vi "03 - 2D Picture.vi"() -> ()   [LabVIEW 2019]
uses:
  Shared/Direction--enum.ctl
  Shared/Selection--picture ring.ctl
  Shared/Pen Operation--enum.ctl
  <vilib>/Utility/cursorutil.llb/Set Cursor (Icon Pict).vi
  Grassfire 2D/Grassfire 2D.lvclass
  Grassfire/Grassfire.lvclass
  Shared/Shared.lvlib
panel:
  in  "Zoom":sgl(slide) scale=1.0..5.0
  in  "Tab Control":enum32{"Edit", "Solution"}(tab)
  in  "Tool":enum32{"Erase", "Pen", "Start", "End"}(radio)
  out "Maze":picture
  in  "Load File":bool
  in  "Save File":bool
  in  "Preset 1":bool
  in  "Pen Color":u32(colorbox)=15671808
  in  "Select Pen Attributes":T1={"Width"=6, "Style"=enum."Solid"} {"Width" scale=1.0..5.0}
  in  "Clear":bool
  in  "Selection":T2
  in  "Pen":T3
  in  "Calculate":bool
  in  "Heading":T4=enum."Down"
  out "Maze Solution":picture
  out "ms":u32
  out "Directions":T4[](array[typedef])
  out "Valid":bool
  in  "Calculate using Class in Maps":bool
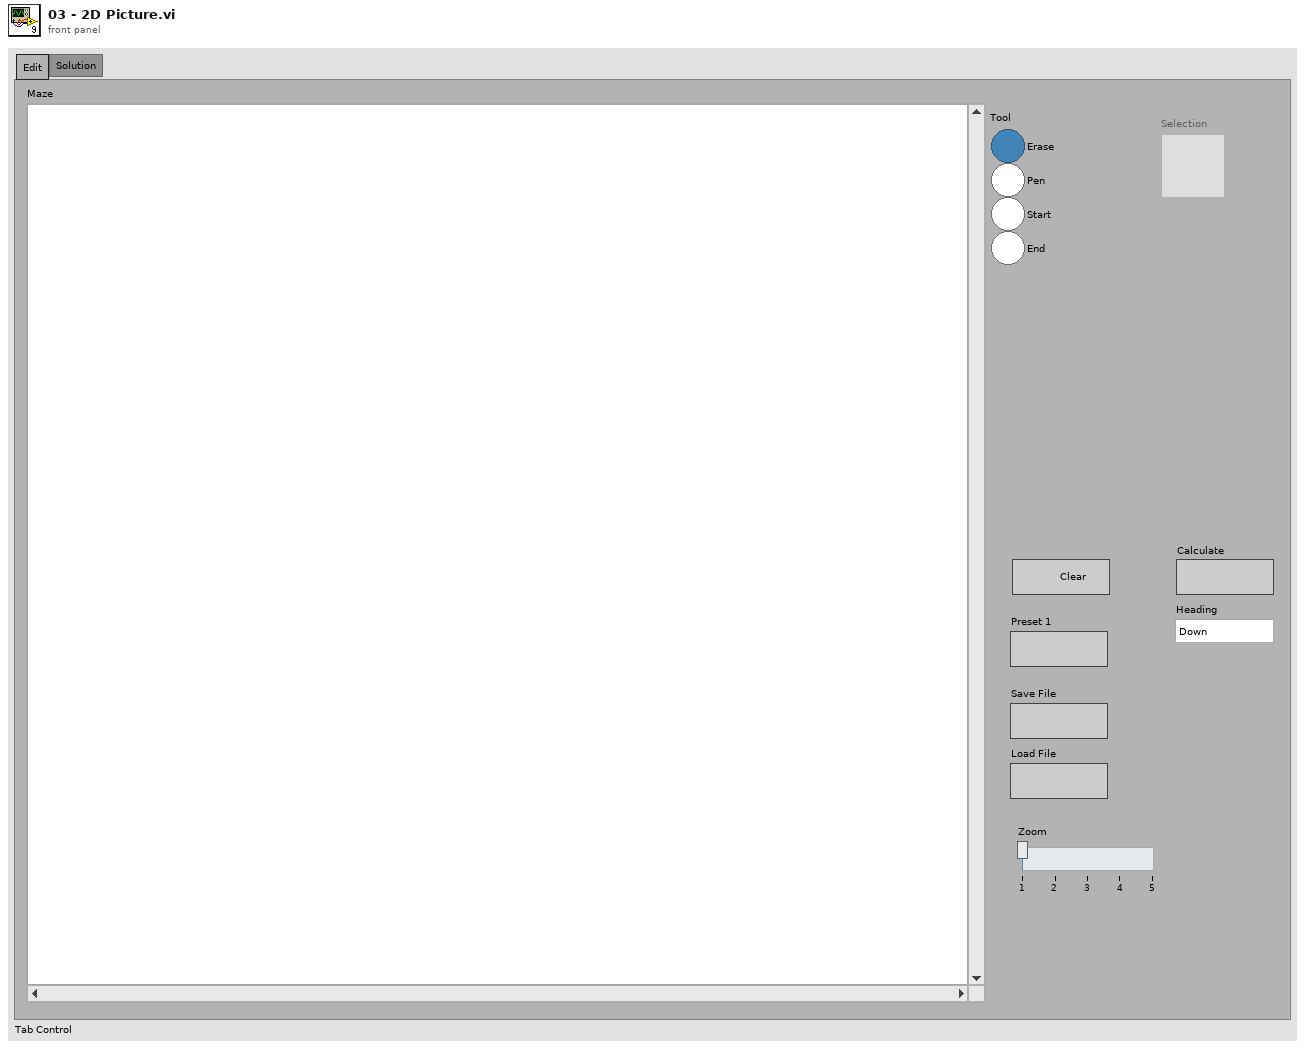
[diagram p1: front panel]
types:
  T1 = cluster{"Width":u16, "Style":enum32{"Solid", "Dash", "Dot", "DashDot", "DashDotDot"}}
  T2 = typedef "Shared.lvlib/Selection--picture ring.ctl" = i64
  T3 = typedef "Shared.lvlib/Pen Operation--enum.ctl" = enum32{"Point", "Free", "Straight Line", "Rectangle"}
  T4 = typedef "Shared.lvlib/Direction--enum.ctl" = enum16{"<Unknown>", "Right", "Down", "Left", "Up"}
  T5 = enum32{"Solid", "Dash", "Dot", "DashDot", "DashDotDot"}
  T6 = typedef "LVMouseTypeDef.ctl" = cluster{"Mouse Position":cluster{"X":i32, "Y":i32}, "Mouse Modifiers":cluster{"Button Down":bool, "Shift Mod":bool, "Menu Mod":bool, "Option Mod":bool}}
  T7 = typedef "imagedata.ctl" = cluster{"image type":i32, "image depth":i32, "image":u8[], "mask":u8[], "colors":u32[], "Rectangle":cluster{"left":i16, "top":i16, "right":i16, "bottom":i16}}
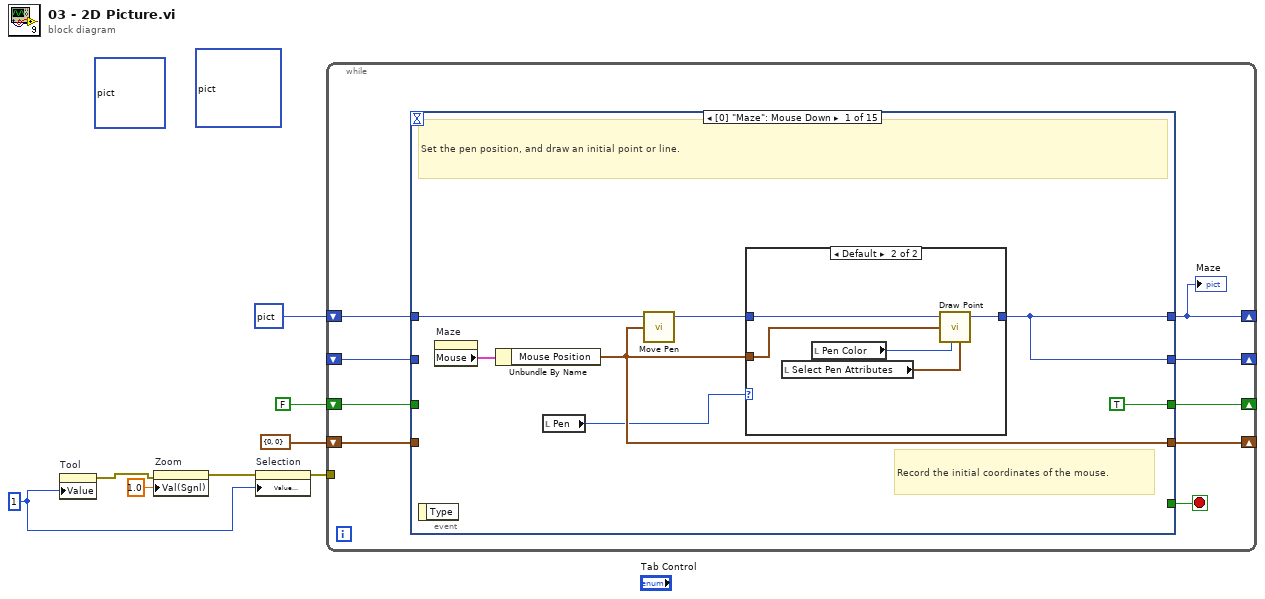
[diagram p0: block diagram]
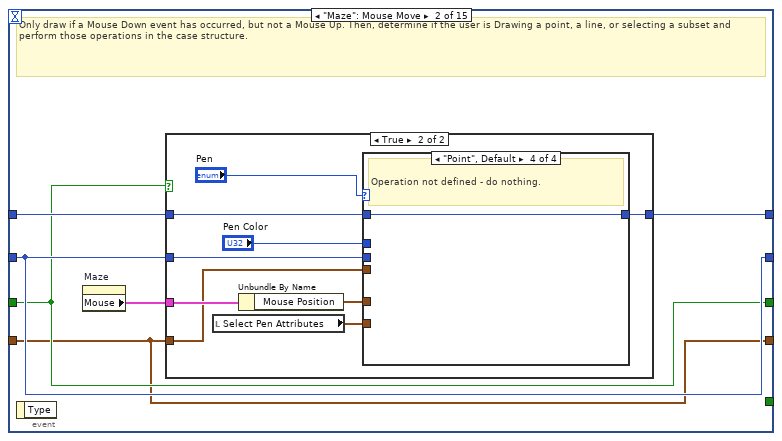
[diagram p3: hidden frame]
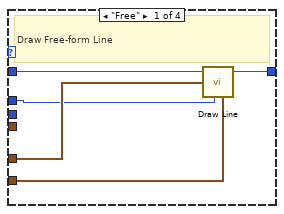
[diagram p5: hidden frame]
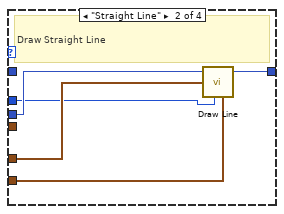
[diagram p6: hidden frame]
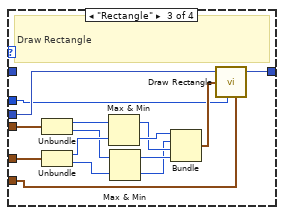
[diagram p7: hidden frame]
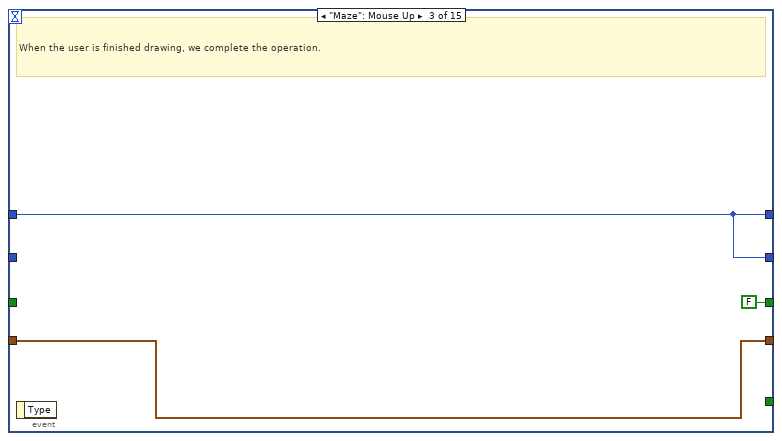
[diagram p8: hidden frame]
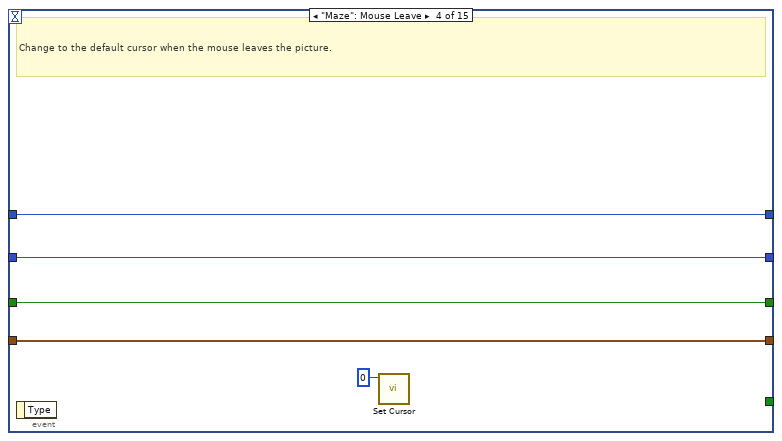
[diagram p9: hidden frame]
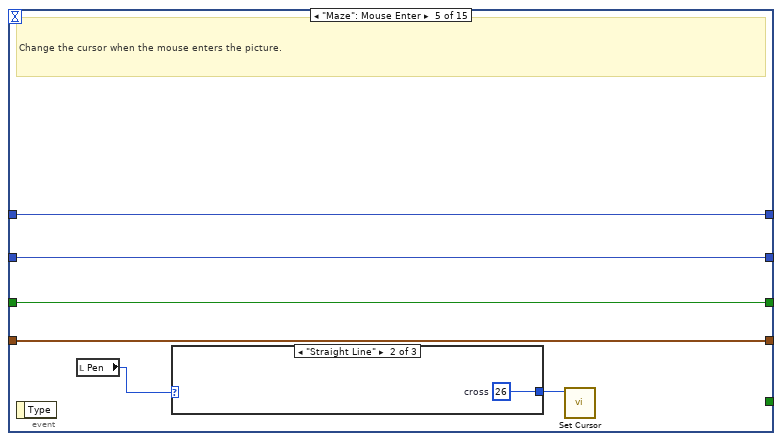
[diagram p10: hidden frame]
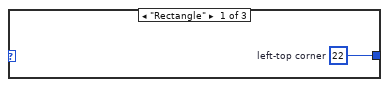
[diagram p11: hidden frame]
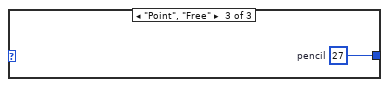
[diagram p12: hidden frame]
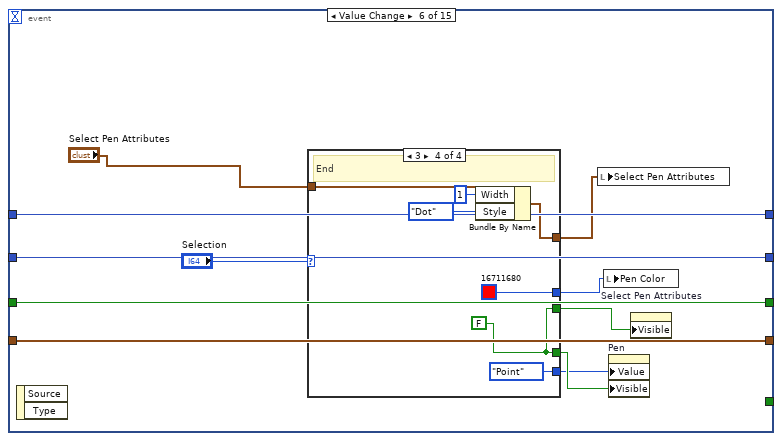
[diagram p13: hidden frame]
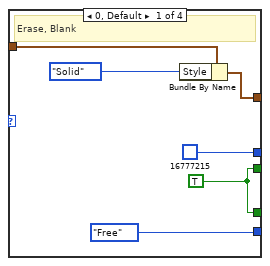
[diagram p14: hidden frame]
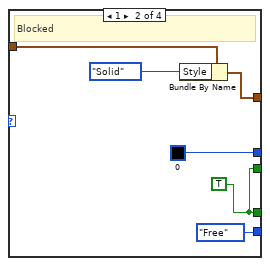
[diagram p15: hidden frame]
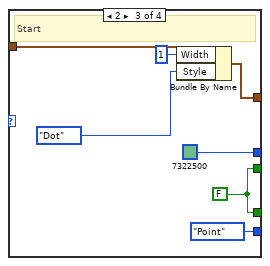
[diagram p16: hidden frame]
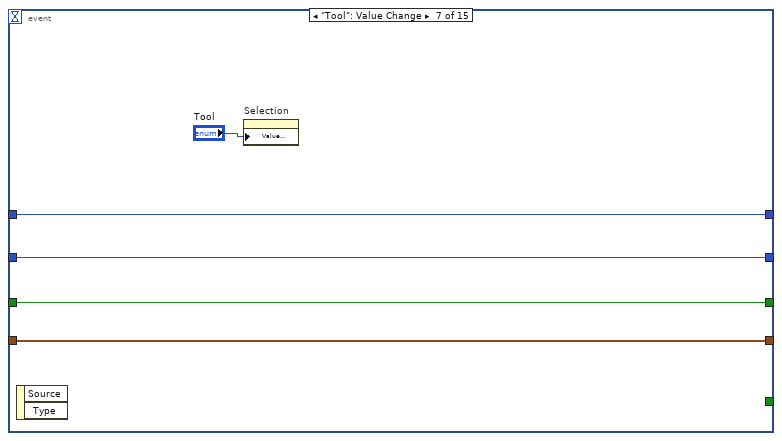
[diagram p17: hidden frame]
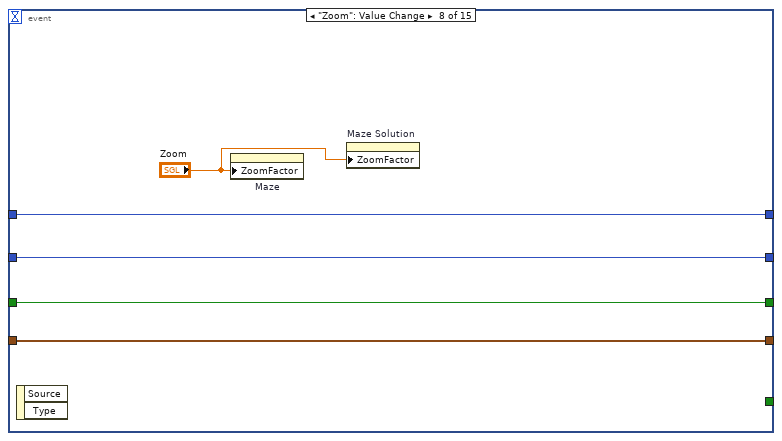
[diagram p18: hidden frame]
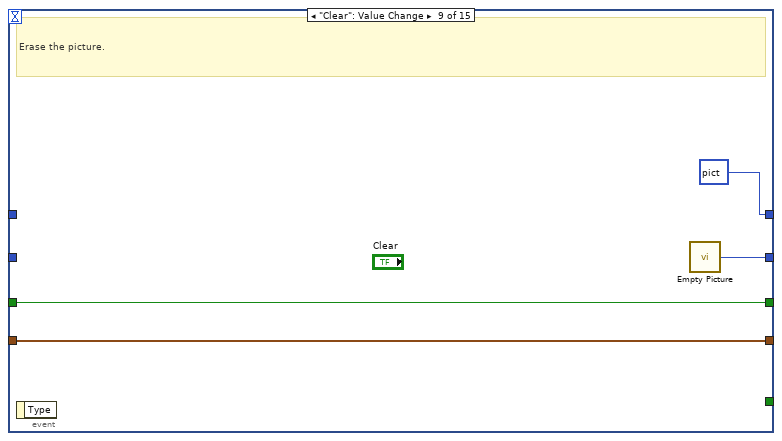
[diagram p19: hidden frame]
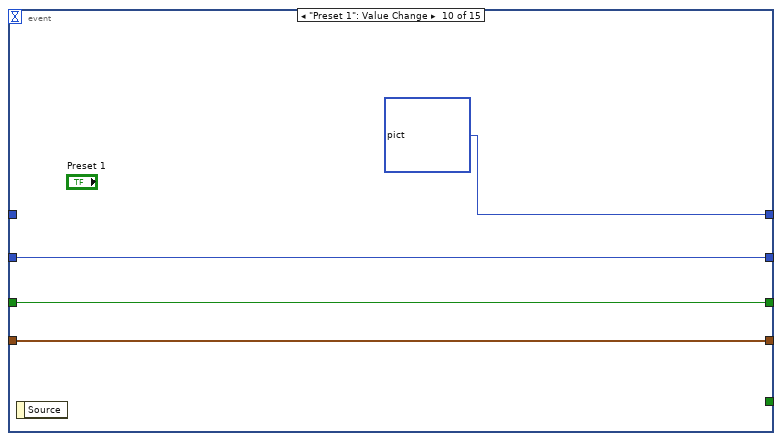
[diagram p20: hidden frame]
diagram:
  (unwired) picture bytes[6048] ("new picture 2")
  (unwired) picture bytes[5924] ("new picture")
  w2 = 1
  n1 = property on="Tool" class="RadioBtnsControl (strict)"("Value"=w2) -> (error out=w3:errorcluster)  [unwired: 2 in, 1 out]
  n2 = property on="Zoom" class="Slide (strict)"(error in=w3, "Val(Sgnl)"=sgl 1.0 ("Value (Signaling)")) -> (error out=w4:errorcluster)  [unwired: 1 in, 1 out]
  n3 = property on="Selection" class="Ring (strict)"(error in=w4, "Value (Signaling)"=w2) -> (error out=w8:errorcluster)  [unwired: 1 in, 1 out]
  n4 = while {
    shift-right: [w16] -> _
    shift-left: _ -> [w15]
    tunnel: w8 -> [_]
    shift-right: [w13] -> _
    shift-left: picture bytes[48] ("Maze") -> [w14]
    shift-right: [w11] -> _
    shift-left: FALSE -> [w12]
    shift-right: [w9] -> _
    shift-left: cluster{"X":i32, "Y":i32} {"X"=0, "Y"=0} ("Mouse Position") -> [w10]
    stop <- w17 stop-if-true
    n5 = event shown="[0] \"Maze\": Mouse Down" {
      selector: _ -> [_ _ _ _ _ _ _ _ _ _ _ _ _ _ _]
      dyn-events: _ -> [_ _ _ _ _ _ _ _ _ _ _ _ _ _ _]
      timeout: _ -> [_ _ _ _ _ _ _ _ _ _ _ _ _ _ _]
      tunnel: [_ _ _ _ _ _ _ _ _ _ _ _ _ _ w198] -> w17
      tunnel: [w21 w35 w75 w79 w85 w100 w131 w136 picture bytes[48] ("Maze") picture bytes[13628] ("Maze") w147 w153 w160 w182 w202] -> w13
      tunnel: w14 -> [w23 w34 w75 w79 w85 w100 w131 w136 _ _ w147 w155 w160 w182 w202]
      tunnel: [w21 w33 w75 w80 w86 w99 w130 w135 w140 w144 w150 w158 w178 w197 w201] -> w16
      tunnel: w15 -> [_ w33 _ w80 w86 w99 w130 w135 _ w144 w150 w158 w178 w197 w201]
      tunnel: w12 -> [_ w32 _ w77 w83 w98 w129 w134 w139 w143 w149 w157 w177 w196 w200]
      tunnel: [TRUE w32 FALSE w77 w83 w98 w129 w134 w139 w143 w149 w157 w177 w196 w200] -> w11
      tunnel: w10 -> [_ w31 w73 w76 w82 w97 w128 w133 w138 w142 w148 w156 w176 w195 w199]
      tunnel: [w19 w31 w73 w76 w82 w97 w128 w133 w138 w142 w148 w156 w176 w195 w199] -> w9
      event "Maze": Mouse Down {
        # "Record the initial coordinates of the mouse."
        # "Set the pen position, and draw an initial point or line."
        n6 = event-data() -> ()  [unwired: 1 in, 1 out]
        n7 = property on="Maze" class="Pict"() -> ("Mouse"=w24:T6)  [unwired: 2 in, 2 out]
        n8 = Unbundle By Name(w24) -> ("Mouse Position"=w19:cluster{"X":i32, "Y":i32})
        n9 = local read "Pen"() -> (w18:T3)
        n10 = call <vilib>:"Move Pen.vi"("new position"=w19, "picture"=w23) -> ("new picture"=w22:picture)  [unwired: 3 in]
        n11 = case shown="Default" w18 {
          tunnel: w22 -> [w25 w30]
          tunnel: [w25 w29] -> w21
          tunnel: w19 -> [_ w28]
          frame "Rectangle" {
          }
          frame Default {
            n12 = local read "Select Pen Attributes"() -> (w26:T1)
            n13 = local read "Pen Color"() -> (w27:u32)
            n14 = call <vilib>:"Draw Point.vi"("picture"=w30, "point(x,y)"=w28, "color(black)"=w27, "pen"=w26) -> ("new picture"=w29:picture)  [unwired: 5 in]
          }
        }
      }
      event "Maze": Mouse Move {
        # "Only draw if a Mouse Down event has occurred, but not a Mouse Up. Then, determine if the user is Drawing a point, a line, or selecting a subset and perform those operations in the case structure."
        n15 = event-data() -> ()  [unwired: 1 in, 1 out]
        n16 = property on="Maze" class="Pict"() -> ("Mouse"=w36:T6)  [unwired: 2 in, 2 out]
        n17 = case shown="True" w32 {
          tunnel: w34 -> [w37 w46]
          tunnel: w36 -> [_ w45]
          tunnel: [w37 w43] -> w35
          tunnel: w33 -> [_ w42]
          tunnel: w31 -> [_ w41]
          frame False {
          }
          frame True {
            n18 = local read "Select Pen Attributes"() -> (w40:T1)
            n19 = Unbundle By Name(w45) -> ("Mouse Position"=w44:cluster{"X":i32, "Y":i32})
            n20 = case shown="\"Point\", Default" "Pen" {
              tunnel: w46 -> [w49 _ _ w72]
              tunnel: w41 -> [_ _ w70 _]
              tunnel: w44 -> [w50 w55 w71 _]
              tunnel: [w51 w56 w68 w72] -> w43
              tunnel: w42 -> [_ w54 w60 _]
              tunnel: w40 -> [w47 w53 w59 _]
              tunnel: "Pen Color" -> [w48 w52 w58 _]
              frame "Free" {
                # "Draw Free-form Line"
                n21 = call <vilib>:"Draw Line.vi"("picture"=w49, "end point"=w50, "color(black)"=w48, "pen"=w47) -> ("new picture"=w51:picture)  [unwired: 5 in]
              }
              frame "Straight Line" {
                # "Draw Straight Line"
                n22 = call <vilib>:"Draw Line.vi"("picture"=w54, "end point"=w55, "color(black)"=w52, "pen"=w53) -> ("new picture"=w56:picture)  [unwired: 5 in]
              }
              frame "Rectangle" {
                # "Draw Rectangle"
                n23 = Unbundle(w70) -> ("X"=w67:i32, "Y"=w57:i32)
                n24 = Unbundle(w71) -> ("X"=w66:i32, "Y"=w63:i32)
                n25 = Max & Min(x=w67, y=w66) -> (max(x,y)=w64:i32, min(x,y)=w65:i32)
                n26 = Max & Min(x=w57, y=w63) -> (max(x,y)=w62:i32, min(x,y)=w61:i32)
                n27 = Bundle(w65, w61, w64, w62) -> (w69:cluster{i32, i32, i32, i32})  [unwired: 1 in]
                n28 = call <vilib>:"Draw Rectangle.vi"("picture"=w60, "rect"=w69, "color(black)"=w58, "pen"=w59) -> ("new picture"=w68:picture)  [unwired: 5 in]
              }
              frame "Point", Default {
                # "Operation not defined - do nothing."
              }
            }
          }
        }
      }
      event "Maze": Mouse Up {
        # "When the user is finished drawing, we complete the operation."
        n29 = event-data() -> ()  [unwired: 1 in, 1 out]
      }
      event "Maze": Mouse Leave {
        # "Change to the default cursor when the mouse leaves the picture."
        n30 = event-data() -> ()  [unwired: 1 in, 1 out]
        n31 = call-poly <vilib>:"Set Cursor.vi"("icon"=u16 0) -> ()  [unwired: 9 in, 2 out]
      }
      event "Maze": Mouse Enter {
        # "Change the cursor when the mouse enters the picture."
        n32 = event-data() -> ()  [unwired: 1 in, 1 out]
        n33 = local read "Pen"() -> (w81:T3)
        n34 = case shown="\"Straight Line\"" w81 {
          tunnel: [w87 w88 w89] -> w84
          frame "Rectangle" {
            w87 = u16 22  # left-top corner
          }
          frame "Straight Line" {
            w88 = u16 26  # cross
          }
          frame "Point", "Free" {
            w89 = u16 27  # pencil
          }
        }
        n35 = call-poly <vilib>:"Set Cursor.vi"("icon"=w84) -> ()  [unwired: 9 in, 2 out]
      }
      event Value Change {
        n36 = event-data() -> ()  [unwired: 1 in, 2 out]
        n37 = case shown="3" "Selection" {
          tunnel: [w104 w111 w117 w124] -> w95
          tunnel: [u32 16777215 ("Pen Color") u32 0 ("Pen Color") u32 7322500 ("Pen Color") u32 16711680 ("Pen Color")] -> w94
          tunnel: "Select Pen Attributes" -> [w105 w112 w118 w125]
          tunnel: [w101 w107 w113 w120] -> w93
          tunnel: [w101 w107 w113 w120] -> w91
          tunnel: [Pen_Operation--enum."Free" ("Pen") Pen_Operation--enum."Free" ("Pen") Pen_Operation--enum."Point" ("Pen") Pen_Operation--enum."Point" ("Pen")] -> w92
          frame 0, Default {
            w101 = TRUE
            # "Erase, Blank"
            n38 = Bundle By Name(cluster=w105, "Style"=T5."Solid") -> (w104:T1)
          }
          frame 1 {
            w107 = TRUE
            # "Blocked"
            n39 = Bundle By Name(cluster=w112, "Style"=T5."Solid") -> (w111:T1)
          }
          frame 2 {
            w113 = FALSE
            # "Start"
            n40 = Bundle By Name(cluster=w118, "Width"=u16 1, "Style"=T5."Dot") -> (w117:T1)
          }
          frame 3 {
            w120 = FALSE
            # "End"
            n41 = Bundle By Name(cluster=w125, "Width"=u16 1, "Style"=T5."Dot") -> (w124:T1)
          }
        }
        n42 = local write "Select Pen Attributes"(w95) -> ()
        n43 = local write "Pen Color"(w94) -> ()
        n44 = property on="Pen" class="RadioBtnsControl (strict)"("Value"=w92, "Visible"=w93) -> ()  [unwired: 2 in, 2 out]
        n45 = property on="Select Pen Attributes" class="Clust (strict)"("Visible"=w91) -> ()  [unwired: 2 in, 2 out]
      }
      event "Tool": Value Change {
        n46 = event-data() -> ()  [unwired: 1 in, 2 out]
        n47 = property on="Selection" class="Ring (strict)"("Value (Signaling)"="Tool") -> ()  [unwired: 2 in, 2 out]
      }
      event "Zoom": Value Change {
        n48 = event-data() -> ()  [unwired: 1 in, 2 out]
        n49 = property on="Maze" class="Pict"("ZoomFactor"="Zoom") -> ()  [unwired: 2 in, 2 out]
        n50 = property on="Maze Solution" class="Pict"("ZoomFactor"="Zoom") -> ()  [unwired: 2 in, 2 out]
      }
      event "Clear": Value Change {
        # "Erase the picture."
        n51 = event-data() -> ()  [unwired: 1 in, 1 out]
        n52 = call "Empty Picture"() -> ("empty picture"=w140:picture)
      }
      event "Preset 1": Value Change {
        n53 = event-data() -> ()  [unwired: 1 in, 1 out]
      }
      event "Save File": Value Change {
        n54 = event-data() -> ()  [unwired: 1 in, 1 out]
        n55 = call <vilib>:"Picture to Pixmap.vi"("picture"=w147) -> ("image data"=w146:T7)  [unwired: 9 in, 1 out]
        n56 = call <vilib>:"Write PNG File.vi"("image data"=w146) -> ("error out"=w145:errorcluster)  [unwired: 9 in, 1 out]
        n57 = call <vilib>:"Clear Errors.vi"("error in (no error)"=w145) -> ()  [unwired: 5 in, 2 out]
      }
      event "Load File": Value Change {
        n58 = event-data() -> ()  [unwired: 1 in, 1 out]
        n59 = call <vilib>:"Read PNG File.vi"() -> ("error out"=w151:errorcluster, "image data"=w152:T7)  [unwired: 9 in, 1 out]
        n60 = call <vilib>:"Draw Flattened Pixmap.vi"("image data"=w152) -> ("new picture"=w154:picture)  [unwired: 8 in]
        n61 = Select(t=w155, s=w151, f=w154) -> (s? t:f=w153:picture)
      }
      event "Calculate": Value Change {
        n62 = event-data() -> ()  [unwired: 1 in, 1 out]
        n63 = call <userlib>:"Tick Count (ms)__ogtk.vi"() -> ("error out"=w173:errorcluster, "millisecond timer value"=w172:u32)  [unwired: 10 in]
        n64 = call "Initialise Picture.vi"("error in (no error)"=w173, "picture"=w160) -> ("error out"=w168:errorcluster, "Valid"=→"Valid":bool, "Grassfire 2D out"=w161:refnum<class "Grassfire 2D.lvclass">)  [unwired: 7 in]
        n65 = call-dynamic "Calculate Distances.vi"("error in (no error)"=w168, "Grassfire 2D In"=w161) -> ("error out"=w169:errorcluster, "Grassfire 2D Out"=w162:refnum<class "Grassfire 2D.lvclass">)  [unwired: 8 in]
        n66 = call-dynamic "Calculate Directions.vi"("error in (no error)"=w169, "Heading"="Heading", "Grassfire 2D In"=w162) -> ("error out"=w170:errorcluster, "Directions"=→"Directions":T4[], "Grassfire 2D Out"=w166:refnum<class "Grassfire 2D.lvclass">)  [unwired: 6 in]
        n67 = call "Get Picture Solution.vi"("error in (no error)"=w170, "Grassfire 2D In"=w166) -> ("error out"=w174:errorcluster, "2D Picture"=→"Maze Solution":picture)  [unwired: 7 in, 1 out]
        n68 = call <userlib>:"Tick Count (ms)__ogtk.vi"("error in (no error)"=w174) -> ("millisecond timer value"=w171:u32)  [unwired: 9 in, 1 out]
        n69 = Subtract(x=w171, y=w172) -> (x-y=→"ms":u32)
        n70 = local write "Tab Control"(enum32{"Edit", "Solution"}."Solution" ("Tab Control")) -> ()
      }
      event "Calculate using Class in Maps": Value Change {
        n71 = event-data() -> ()  [unwired: 1 in, 1 out]
        n72 = call <userlib>:"Tick Count (ms)__ogtk.vi"() -> ("error out"=w190:errorcluster, "millisecond timer value"=w193:u32)  [unwired: 10 in]
        n73 = call "Set 2D Picture.vi"("error in (no error)"=w190, "picture"=w182) -> ("error out"=w181:errorcluster, "Valid"=w185:bool, "Grassfire out"=w183:refnum<class "Grassfire.lvclass">)  [unwired: 7 in]
        n74 = local read "Heading"() -> (w186:T4)
        n75 = local write "Valid"(w185) -> ()
        n76 = call-dynamic "Calculate Distances with set.vi"("error in (no error)"=w181, "Grassfire in"=w183) -> ("error out"=w180:errorcluster, "Grassfire out"=w184:refnum<class "Grassfire.lvclass">)  [unwired: 8 in]
        n77 = call-dynamic "Calculate Directions.vi"("error in (no error)"=w180, "Heading"=w186, "Grassfire in"=w184) -> ("error out"=w179:errorcluster, "Directions"=w187:T4[], "Grassfire out"=w188:refnum<class "Grassfire.lvclass">)  [unwired: 6 in]
        n78 = call-dynamic "Get 2D Picture from Map.vi"("error in (no error)"=w179, "Grassfire in"=w188) -> ("error out"=w191:errorcluster, "2D Picture"=w189:picture)  [unwired: 7 in, 1 out]
        n79 = local write "Directions"(w187) -> ()
        n80 = local write "Maze Solution"(w189) -> ()
        n81 = call <userlib>:"Tick Count (ms)__ogtk.vi"("error in (no error)"=w191) -> ("millisecond timer value"=w192:u32)  [unwired: 9 in, 1 out]
        n82 = Subtract(x=w192, y=w193) -> (x-y=w194:u32)
        n83 = local write "ms"(w194) -> ()
      }
      event Panel Close? {
        w198 = TRUE ("Discard?")
        n84 = event-data() -> ()  [unwired: 1 in, 1 out]
        n85 = event-data("Discard?"=w198) -> ()  [unwired: 1 in, 1 out]
      }
    }
    "Maze" <- w13
  }
